vi "Read File.vi"(8 "error in (no error)":errorcluster, 10 "Path in":path, 11 "Reflective Memory File in":refnum<class "Reflective Memory File.lvclass">) -> (0 "error out":errorcluster, 2 "SysDef":T1 {"Tree"."Properties"."Type" items=["K_STRING", "K_BOOL", "K_I32", "K_U32", "K_DOUBLE", "K_U64", "K_VARIANT", "K_DEPENDENTFILE", "K_DEPENDENTNODE", "K_DATASOURCENODE", "K_U16", "K_DBLARR", "K_U32ARR", "K_I32ARR", "K_STRINGARR", "K_DICTIONARY", "K_DICTIONARYARR"]})   [LabVIEW 2017, in "RefMem DMA Custom Device.lvlib" / "Reflective Memory File.lvclass"]
uses:
  RefMem DMA Configuration.llb/Reflective Memory File.lvclass
  RefMem DMA Configuration.llb/SysDef.Export.ctl
  RefMem DMA Configuration.llb/TreeItem.ctl
  RefMem DMA Configuration.llb/TreeItem.Info.ctl
  RefMem DMA Configuration.llb/Custom Device Channel.ctl
  RefMem DMA Configuration.llb/Custom Device Channel Type.ctl
  RefMem DMA Configuration.llb/Custom Device Waveform.ctl
  RefMem DMA Configuration.llb/Custom Device Waveform DataType.ctl
  RefMem DMA Configuration.llb/TreeItem.Property.ctl
  RefMem DMA Custom Device/Data Channel Type.ctl
  RefMem DMA Custom Device/Global.vi
  RefMem DMA Configuration.llb/Custom Device API.lvlib
  RefMem DMA Configuration.llb/Advanced System Definition.lvlib
  RefMem DMA Configuration.llb/RefMem DMA Custom Device.lvlib
panel:
  out "deleted portion":string[](array[string])
  out "array w/ subset deleted":string[][](array[string])
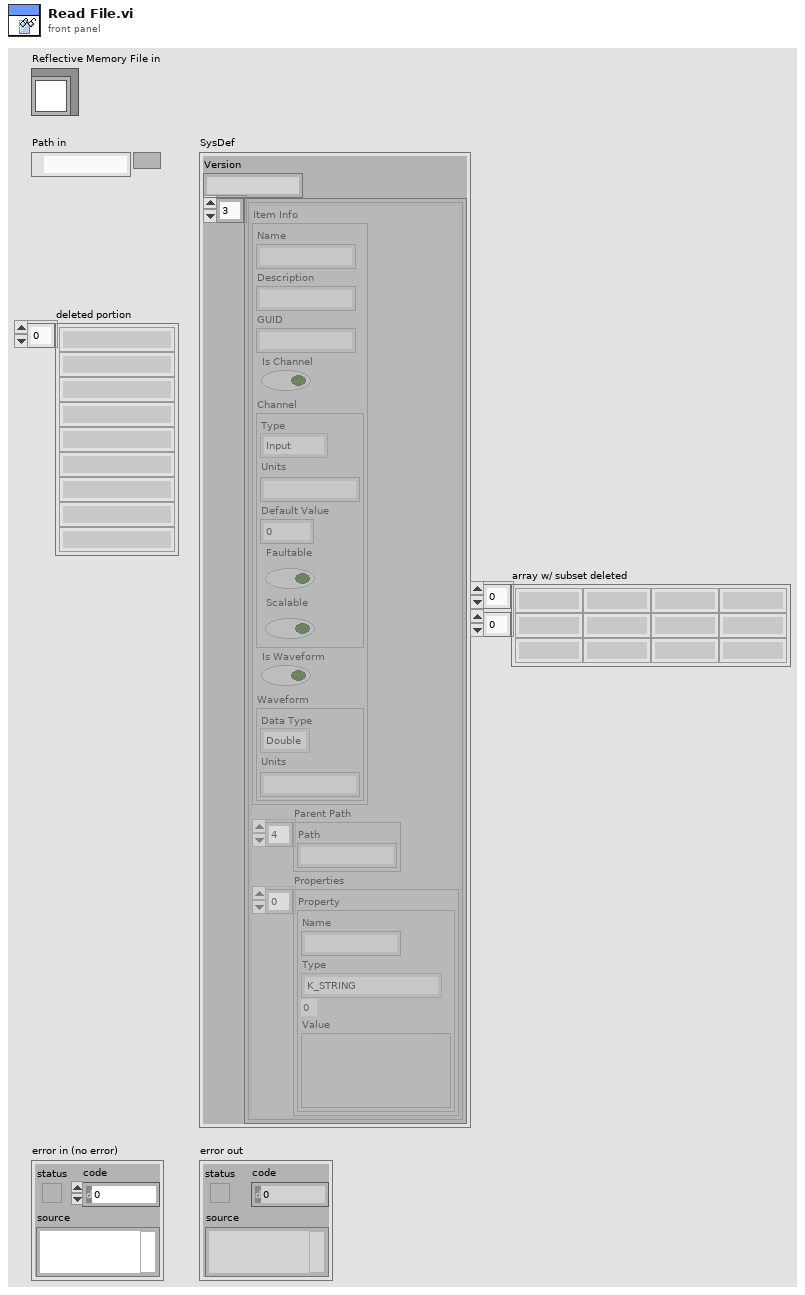
[diagram p1: front panel]
types:
  T1 = typedef "Advanced System Definition.lvlib/SysDef.Export.ctl" = cluster{"Version":string, "Tree":T2[]}
  T2 = typedef "Advanced System Definition.lvlib/TreeItem.ctl" = cluster{"Item Info":T3, "Parent Path":string[], "Properties":T8[]}
  T3 = typedef "Advanced System Definition.lvlib/TreeItem.Info.ctl" = cluster{"Name":string, "Description":string, "GUID":string, "Is Channel":bool, "Channel":T4, "Is Waveform":bool, "Waveform":T6}
  T4 = typedef "Custom Device API.lvlib/Custom Device Channel.ctl" = cluster{"Type":T5, "Units":string, "Default Value":dbl, "Faultable":bool, "Scalable":bool}
  T5 = typedef "Custom Device API.lvlib/Custom Device Channel Type.ctl" = enum16{"Input", "Output"}
  T6 = typedef "Custom Device API.lvlib/Custom Device Waveform.ctl" = cluster{"Data Type":T7, "Units":string}
  T7 = typedef "Custom Device API.lvlib/Custom Device Waveform DataType.ctl" = enum16{"Double", "Complex Double"}
  T8 = typedef "Advanced System Definition.lvlib/TreeItem.Property.ctl" = cluster{"Name":string, "Type":i32, "Value":variant}
  T9 = typedef "RefMem DMA Custom Device.lvlib/Data Channel Type.ctl" = enum16{"Read", "Write"}
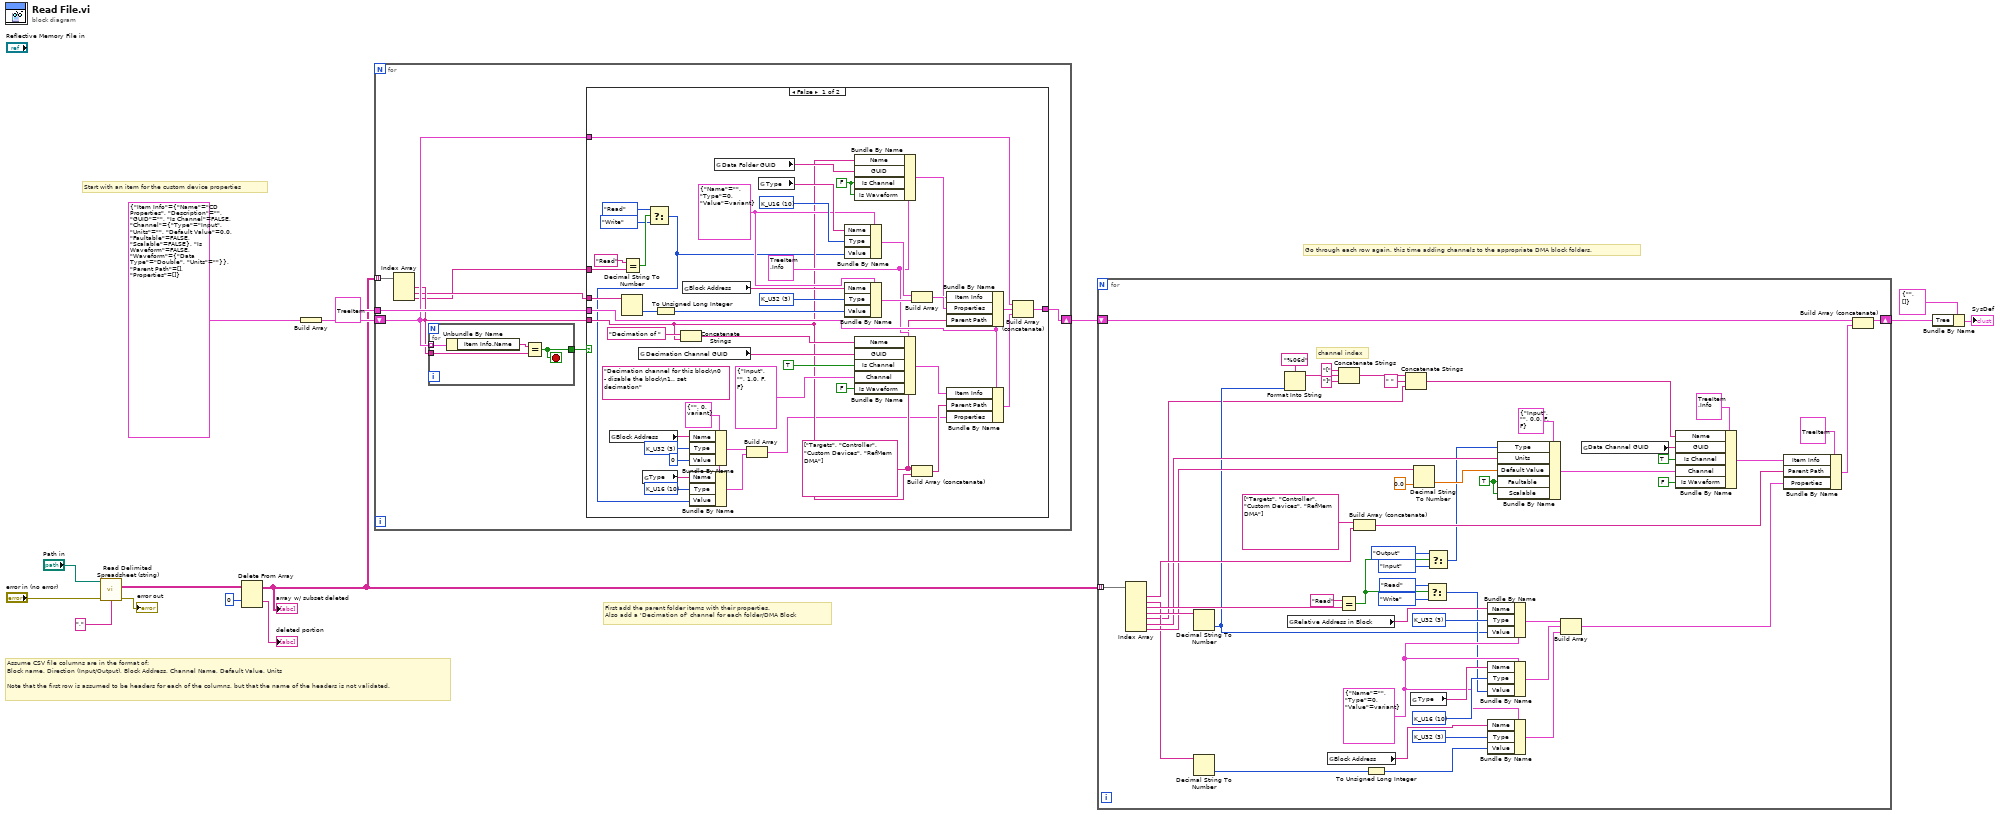
[diagram p0: block diagram]
diagram:
  # "Go through each row again, this time adding channels to the appropriate DMA block folders."
  # "First add the parent folder items with their properties.\nAlso add a 'Decimation of' channel for each folder/DMA Block"
  # "Assume CSV file columns are in the format of:\nBlock name, Direction (Input/Output), Block Address, Channel Name, Default Value, Units\n\nNote that the first row is assumed to be headers for each of the columns, but that the name of the headers is not validated."
  # "Start with an item for the custom device properties"
  n1 = call "Read Delimited Spreadsheet (string).vi"("file path (dialog if empty)"="Path in", "error in (no error)"="error in (no error)", "delimiter (\\t)"="," ("delimiter (\\t)")) -> ("all rows"=w14:string[][], "error out"=→"error out":errorcluster)  [unwired: 7 in, 4 out]
  n2 = Delete From Array(array=w14, index (row)=0) -> (deleted portion=→"deleted portion":string[], array with subset deleted=w1:string[][])  [unwired: 2 in]
  "array w/ subset deleted" <- w1
  n3 = Build Array(T2 {"Item Info"={"Name"="CD Properties", "Description"="", "GUID"="", "Is Channel"=FALSE, "Channel"={"Type"=enum."Input", "Units"="", "Default Value"=0.0, "Faultable"=FALSE, "Scalable"=FALSE}, "Is Waveform"=FALSE, "Waveform"={"Data Type"=enum."Double", "Units"=""}}, "Parent Path"=[], "Properties"=[]} ("TreeItem")) -> (w2:T2[])
  n4 = for {
    tunnel: w1 -> [w22] mode=indexing
    shift-right: [w21] -> w6
    shift-left: w2 -> [w20]
    tunnel: T2 {"Item Info"={"Name"="", "Description"="", "GUID"="", "Is Channel"=FALSE, "Channel"={"Type"=enum."Input", "Units"="", "Default Value"=0.0, "Faultable"=FALSE, "Scalable"=FALSE}, "Is Waveform"=FALSE, "Waveform"={"Data Type"=enum."Double", "Units"=""}}, "Parent Path"=[], "Properties"=[]} ("TreeItem") -> [w23]
    n5 = Index Array(array=w22) -> (element #1=w19:string, element #2=w17:string, element #3=w16:string)  [unwired: 3 in]
    n6 = for {
      tunnel: w20 -> [w73] mode=indexing
      tunnel: w19 -> [w71]
      tunnel: [w70] -> w18
      stop <- w70 stop-if-true
      n7 = Unbundle By Name(w73) -> ("Item Info.Name"=w72:string)
      n8 = Equal?(x=w72, y=w71) -> (x = y?=w70:bool)
    }
    n9 = case shown="False" w18 {
      tunnel: w23 -> [w44 _]
      tunnel: w16 -> [w64 _]
      tunnel: [w57 w69] -> w21
      tunnel: w17 -> [w56 _]
      tunnel: w20 -> [w49 w69]
      tunnel: w19 -> [w29 _]
      frame False {
        w33 = 10 items=["K_STRING", "K_BOOL", "K_I32", "K_U32", "K_DOUBLE", "K_U64", "K_VARIANT", "K_DEPENDENTFILE", "K_DEPENDENTNODE", "K_DATASOURCENODE", "K_U16", "K_DBLARR", "K_U32ARR", "K_I32ARR", "K_STRINGARR", "K_DICTIONARY", "K_DICTIONARYARR"] ("Type")
        w35 = 3 items=["K_STRING", "K_BOOL", "K_I32", "K_U32", "K_DOUBLE", "K_U64", "K_VARIANT", "K_DEPENDENTFILE", "K_DEPENDENTNODE", "K_DATASOURCENODE", "K_U16", "K_DBLARR", "K_U32ARR", "K_I32ARR", "K_STRINGARR", "K_DICTIONARY", "K_DICTIONARYARR"] ("Type")
        w31 = T8 {"Name"="", "Type"=0, "Value"=variant} ("Property")
        w38 = string[] ["Targets", "Controller", "Custom Devices", "RefMem DMA"]
        (unwired) "Decimation channel for this block\n0 - disable the block\n1.. set decimation" ("Section Name")
        w52 = 3 items=["K_STRING", "K_BOOL", "K_I32", "K_U32", "K_DOUBLE", "K_U64", "K_VARIANT", "K_DEPENDENTFILE", "K_DEPENDENTNODE", "K_DATASOURCENODE", "K_U16", "K_DBLARR", "K_U32ARR", "K_I32ARR", "K_STRINGARR", "K_DICTIONARY", "K_DICTIONARYARR"] ("Type")
        w65 = 10 items=["K_STRING", "K_BOOL", "K_I32", "K_U32", "K_DOUBLE", "K_U64", "K_VARIANT", "K_DEPENDENTFILE", "K_DEPENDENTNODE", "K_DATASOURCENODE", "K_U16", "K_DBLARR", "K_U32ARR", "K_I32ARR", "K_STRINGARR", "K_DICTIONARY", "K_DICTIONARYARR"] ("Type")
        w55 = T8 {"Name"="", "Type"=0, "Value"=variant} ("Property")
        w68 = FALSE ("Is Channel")
        w43 = T3 {"Name"="", "Description"="", "GUID"="", "Is Channel"=FALSE, "Channel"={"Type"=enum."Input", "Units"="", "Default Value"=0.0, "Faultable"=FALSE, "Scalable"=FALSE}, "Is Waveform"=FALSE, "Waveform"={"Data Type"=enum."Double", "Units"=""}} ("Item Info")
        n10 = global read "Global.vi" "Block Address"() -> (w36:string)
        n11 = Decimal String To Number(string=w56) -> (number=w51:i32)  [unwired: 2 in, 1 out]
        n12 = Equal?(x="Read", y=w64) -> (x = y?=w62:bool)
        n13 = global read "Global.vi" "Decimation Channel GUID"() -> (w46:string)
        n14 = global read "Global.vi" "Type"() -> (w32:string)
        n15 = Select(t=Data_Channel_Type."Read" ("Type"), s=w62, f=Data_Channel_Type."Write" ("Type")) -> (s? t:f=w28:T9)
        n16 = To Unsigned Long Integer(number=w51) -> (unsigned 32bit integer=w50:u32)
        n17 = Concatenate Strings("Decimation of " ("string"), w29) -> (w47:string)
        n18 = global read "Global.vi" "Block Address"() -> (w53:string)
        n19 = Bundle By Name(cluster=w31, "Name"=w36, "Type"=w35, "Value"=u32 0) -> (w27:T8)
        n20 = Bundle By Name(cluster=w31, "Name"=w32, "Type"=w33, "Value"=w28) -> (w26:T8)
        n21 = global read "Global.vi" "Data Folder GUID"() -> (w67:string)
        n22 = Build Array(w27, w26) -> (w25:T8[])
        n23 = global read "Global.vi" "Type"() -> (w66:string)
        n24 = Bundle By Name(cluster=w55, "Name"=w66, "Type"=w65, "Value"=w28) -> (w61:T8)
        n25 = Bundle By Name(cluster=w55, "Name"=w53, "Type"=w52, "Value"=w50) -> (w54:T8)
        n26 = Bundle By Name(cluster=w43, "Name"=w29, "GUID"=w67, "Is Channel"=w68, "Is Waveform"=w68) -> (w59:T3)
        n27 = Bundle By Name(cluster=w43, "Name"=w47, "GUID"=w46, "Is Channel"=TRUE, "Channel"=T4 {"Type"=enum."Input", "Units"="", "Default Value"=1.0, "Faultable"=FALSE, "Scalable"=FALSE}, "Is Waveform"=FALSE) -> (w24:T3)
        n28 = Build Array(w61, w54) -> (w60:T8[])
        n29 = Build Array (concatenate)(w38, w29) -> (w39:string[])
        n30 = Bundle By Name(cluster=w44, "Item Info"=w59, "Properties"=w60, "Parent Path"=w38) -> (w58:T2)
        n31 = Bundle By Name(cluster=w44, "Item Info"=w24, "Parent Path"=w39, "Properties"=w25) -> (w42:T2)
        n32 = Build Array (concatenate)(w49, w58, w42) -> (w57:T2[])
      }
      frame True {
      }
    }
  }
  n33 = for {
    tunnel: w1 -> [w125] mode=indexing
    shift-right: [w98] -> w5
    shift-left: w6 -> [w97]
    w108 = 10 items=["K_STRING", "K_BOOL", "K_I32", "K_U32", "K_DOUBLE", "K_U64", "K_VARIANT", "K_DEPENDENTFILE", "K_DEPENDENTNODE", "K_DATASOURCENODE", "K_U16", "K_DBLARR", "K_U32ARR", "K_I32ARR", "K_STRINGARR", "K_DICTIONARY", "K_DICTIONARYARR"] ("Type")
    w105 = 3 items=["K_STRING", "K_BOOL", "K_I32", "K_U32", "K_DOUBLE", "K_U64", "K_VARIANT", "K_DEPENDENTFILE", "K_DEPENDENTNODE", "K_DATASOURCENODE", "K_U16", "K_DBLARR", "K_U32ARR", "K_I32ARR", "K_STRINGARR", "K_DICTIONARY", "K_DICTIONARYARR"] ("Type")
    w113 = 3 items=["K_STRING", "K_BOOL", "K_I32", "K_U32", "K_DOUBLE", "K_U64", "K_VARIANT", "K_DEPENDENTFILE", "K_DEPENDENTNODE", "K_DATASOURCENODE", "K_U16", "K_DBLARR", "K_U32ARR", "K_I32ARR", "K_STRINGARR", "K_DICTIONARY", "K_DICTIONARYARR"] ("Type")
    w103 = T8 {"Name"="", "Type"=0, "Value"=variant} ("Property")
    w120 = TRUE ("Faultable")
    # "channel index"
    n34 = Index Array(array=w125) -> (element #1=w115:string, element #2=w87:string, element #3=w90:string, element #4=w91:string, element #5=w76:string, element #6=w89:string, element #7=w88:string)  [unwired: 7 in]
    n35 = Decimal String To Number(string=w91) -> (number=w83:i32)  [unwired: 2 in, 1 out]
    n36 = Decimal String To Number(string=w87) -> (number=w107:i32)  [unwired: 2 in, 1 out]
    n37 = Format Into String(format string="%06d", w83) -> (resulting string=w81:string)  [unwired: 2 in, 1 out]
    n38 = global read "Global.vi" "Relative Address in Block"() -> (w114:string)
    n39 = global read "Global.vi" "Block Address"() -> (w104:string)
    n40 = Concatenate Strings("[" ("string"), w81, "]" ("string")) -> (w78:string)
    n41 = Equal?(x="Read", y=w90) -> (x = y?=w93:bool)
    n42 = Build Array (concatenate)(string[] ["Targets", "Controller", "Custom Devices", "RefMem DMA"], w115) -> (w86:string[])
    n43 = To Unsigned Long Integer(number=w107) -> (unsigned 32bit integer=w106:u32)
    n44 = Concatenate Strings(w78, " " ("string"), w76) -> (w75:string)
    n45 = global read "Global.vi" "Type"() -> (w112:string)
    n46 = Decimal String To Number(string=w88, default (0L)=0.0) -> (number=w79:dbl)  [unwired: 1 in, 1 out]
    n47 = Select(t=Data_Channel_Type."Read" ("Type"), s=w93, f=Data_Channel_Type."Write" ("Type")) -> (s? t:f=w92:T9)
    n48 = Select(t=Custom_Device_Channel_Type."Output" ("Type"), s=w93, f=Custom_Device_Channel_Type."Input" ("Type")) -> (s? t:f=w74:T5)
    n49 = Bundle By Name(cluster=w103, "Name"=w114, "Type"=w113, "Value"=w83) -> (w102:T8)
    n50 = Bundle By Name(cluster=w103, "Name"=w112, "Type"=w108, "Value"=w92) -> (w101:T8)
    n51 = Bundle By Name(cluster=w103, "Name"=w104, "Type"=w105, "Value"=w106) -> (w100:T8)
    n52 = Bundle By Name(cluster=T4 {"Type"=enum."Input", "Units"="", "Default Value"=0.0, "Faultable"=FALSE, "Scalable"=FALSE} ("Channel"), "Type"=w74, "Units"=w89, "Default Value"=w79, "Faultable"=w120, "Scalable"=w120) -> (w118:T4)
    n53 = Build Array(w102, w101, w100) -> (w85:T8[])
    n54 = global read "Global.vi" "Data Channel GUID"() -> (w124:string)
    n55 = Bundle By Name(cluster=T3 {"Name"="", "Description"="", "GUID"="", "Is Channel"=FALSE, "Channel"={"Type"=enum."Input", "Units"="", "Default Value"=0.0, "Faultable"=FALSE, "Scalable"=FALSE}, "Is Waveform"=FALSE, "Waveform"={"Data Type"=enum."Double", "Units"=""}} ("Item Info"), "Name"=w75, "GUID"=w124, "Is Channel"=TRUE, "Channel"=w118, "Is Waveform"=FALSE) -> (w116:T3)
    n56 = Bundle By Name(cluster=T2 {"Item Info"={"Name"="", "Description"="", "GUID"="", "Is Channel"=FALSE, "Channel"={"Type"=enum."Input", "Units"="", "Default Value"=0.0, "Faultable"=FALSE, "Scalable"=FALSE}, "Is Waveform"=FALSE, "Waveform"={"Data Type"=enum."Double", "Units"=""}}, "Parent Path"=[], "Properties"=[]} ("TreeItem"), "Item Info"=w116, "Parent Path"=w86, "Properties"=w85) -> (w99:T2)
    n57 = Build Array (concatenate)(w97, w99) -> (w98:T2[])
  }
  n58 = Bundle By Name(cluster=T1 {"Version"="", "Tree"=[]} ("SysDef"), "Tree"=w5) -> (→"SysDef":T1)
